vi "Read PAQ_memorySizes.vi"(8 "error in (no error)":errorcluster, 11 "FAMM in":refnum<class "FAMM.lvclass">) -> (0 "error out":errorcluster, 2 "Memory Size":i32[](array[numeric]), 3 "FAMM out":refnum<class "FAMM.lvclass">)   [LabVIEW 2020, in "Sgraph_lib_V1.lvlib" / "FAMM.lvclass"]
doc: "Read Size of PAQ memory blocks"
uses:
  FAMM.lvclass
  FAMM.lvclass/FAMM.ctl
  PAQ-memory.lvclass/PAQ-memory.ctl
  PAQ-memory.lvclass
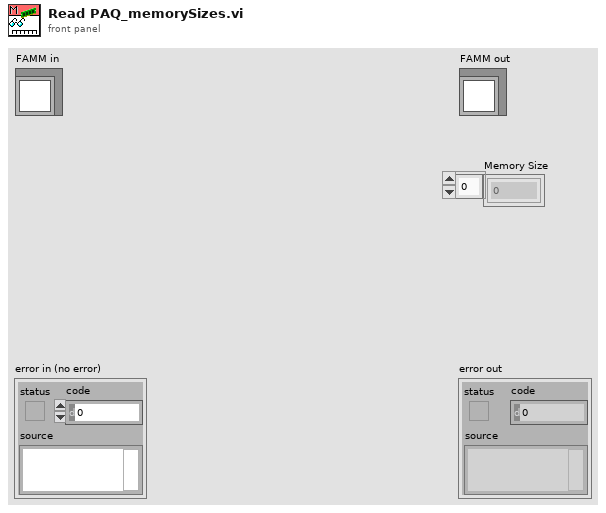
[diagram p1: front panel]
types:
  T1 = typedef "Sgraph_lib_V1.lvlib/FAMM.lvclass/FAMM-attributes.ctl" = cluster{"FAMM_PAQ_Layers":i32, "FAMM_PAQ_resolution":dbl, "PAQ_TAGs":string[], "WAQ_TAGs":string[], "EAQ_TAGs":string[], "All_TAGs":string[], "PAQtagProps":T2[], "WAQtagProps":T2[], "EAQtagProps":T2[], "DBAL_class":refnum<data-value>, "PAQ_memory":refnum<data-value>[], "PAQupdates":timestamp[], "FAMM_Size":cluster{"other":i32, "1day":i32, "1week":i32}, "DatabaseFileExtention":string, "DatabaseSaveRate":dbl, "Database_path":path, "DBAL-Queue":refnum<queue>, "OS_name":string}
  T2 = typedef "Sgraph_lib_V1.lvlib/typedef_com_TagProp.ctl" = cluster{"Description":string, "EngUnits":string, "RangeH":dbl, "RangeL":dbl, "Resolution":i32, "Obsolete":bool, "ChangeDate":timestamp, "ChangeSource":string, "ChangeReason":string, "TagFunc":u32}
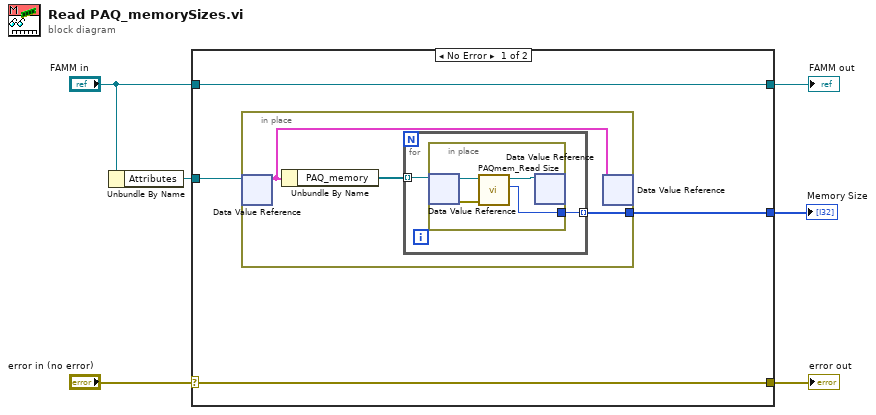
[diagram p0: block diagram]
diagram:
  n1 = Unbundle By Name("FAMM in") -> ("Attributes"=w1:refnum<data-value>)
  n2 = case shown="No Error" "error in (no error)" {
    selector: "error in (no error)" -> [w10 w20]
    tunnel: [w10 w20] -> w5
    tunnel: [w9 w21] -> w4
    tunnel: "FAMM in" -> [w9 w21]
    tunnel: w1 -> [w8 _]
    tunnel: [w7 _] -> w3
    frame No Error {
      n3 = in-place {
        in-place-border: [w13] -> w7
        n4 = in-place-dvr #1(w8) -> (w11:T1)  [unwired: 1 out]
        n5 = Unbundle By Name(w11) -> ("PAQ_memory"=w12:refnum<data-value>[])
        n6 = for {
          tunnel: w12 -> [w15] mode=indexing
          tunnel: [w14] -> w13 mode=indexing
          n7 = in-place {
            in-place-border: [w16] -> w14
            n8 = in-place-dvr #2(w15) -> (w19:refnum<class "PAQ-memory.lvclass">, w18:errorcluster)
            n9 = call "PAQmem_Read Size.vi"("error in (no error)"=w18, "PAQ-memory in"=w19) -> ("Size"=w16:i32, "PAQ-memory out"=w17:refnum<class "PAQ-memory.lvclass">)  [unwired: 7 in, 1 out]
            n10 = in-place-dvr #2(w17) -> ()  [unwired: 2 out]
          }
        }
        n11 = in-place-dvr #1(w11) -> ()  [unwired: 2 out]
      }
    }
    frame Error {
    }
  }
  "error out" <- w5
  "FAMM out" <- w4
  "Memory Size" <- w3
